vi "Write DateTime to Client.vi"(0 "OPC UA client refnum in":T1, 5 "Parent Node In":string, 7 "SubNode ID":string, 11 "error in (no error)":errorcluster, 12 "timestamp (current time)":timestamp) -> (4 "OPC UA client refnum out":T1, 6 "Parent Node Out":string, 15 "error out":errorcluster)   [LabVIEW 2024]
uses:
  <vilib>/OPCUA/controls/OPC UA Client Refnum.ctl
  <vilib>/OPCUA/controls/Write Status.ctl
  <vilib>/OPCUA/controls/NodeId.ctl
  <vilib>/OPCUA/client/Multiple Write DateTime.vi
  <vilib>/OPCUA/NI OPC UA Client.lvlib
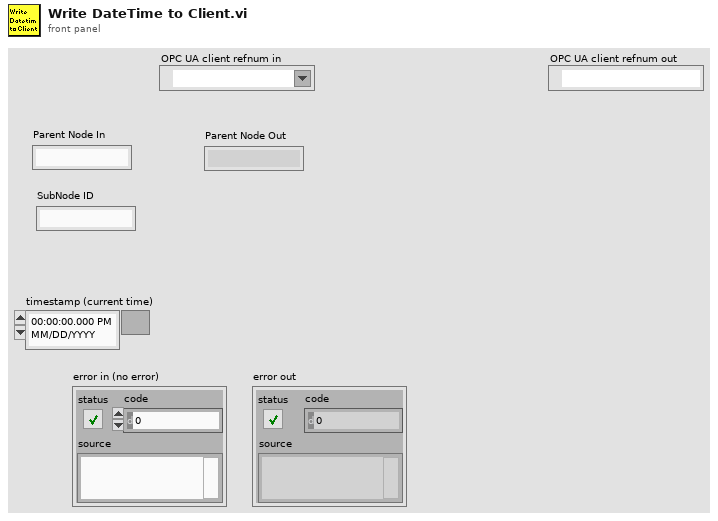
[diagram p1: front panel]
types:
  T1 = typedef "OPC UA Client Refnum.ctl" = refnum<k21>
  T2 = typedef "NodeId.ctl" = string
  T3 = typedef "Write Status.ctl" = u32
  T4 = cluster{"node ID":T2, "value":timestamp, "timestamp (current time)":timestamp, "node status":T3}
  T5 = cluster{"node ID":T2, "value":timestamp, "timestamp (current time)":timestamp, "node status":T3}[]
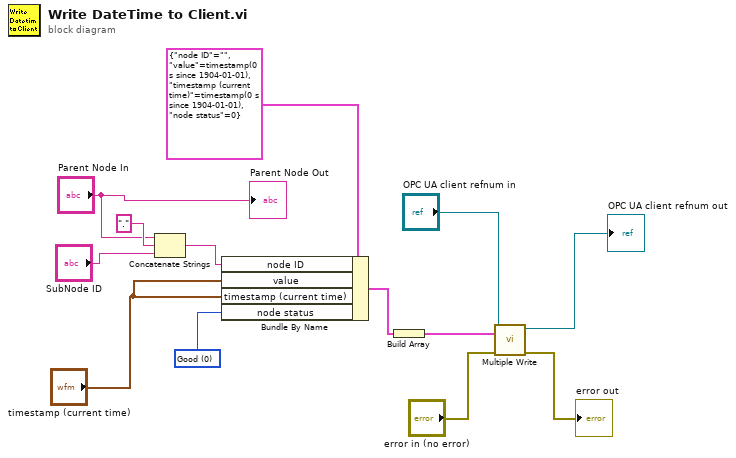
[diagram p0: block diagram]
diagram:
  w6 = T3 0 items=["Good"=0, "Uncertain"=1073741824, "Uncertain_InitialValue"=1083310080, "Uncertain_LastUsableValue"=1083179008, "Uncertain_SensorNotAccurate"=1083375616, "Uncertain_EngineeringUnitsExceeded"=1083441152, "Bad"=2147483648, "Bad_NoCommunication"=2150694912, "Bad_NotReadable"=2151284736, "Bad_NotWritable"=2151350272, "Bad_OutOfRange"=2151415808, "Bad_WaitingForInitialData"=2150760448] ("node status")
  n1 = Concatenate Strings("Parent Node In", ".", "SubNode ID") -> (w5:string)
  n2 = Bundle By Name(cluster=T4 {"node ID"="", "value"=timestamp(0 s since 1904-01-01), "timestamp (current time)"=timestamp(0 s since 1904-01-01), "node status"=0} ("request"), "node ID"=w5, "value"="timestamp (current time)", "timestamp (current time)"="timestamp (current time)", "node status"=w6) -> (w3:T4)
  n3 = Build Array(w3) -> (w2:T5)
  n4 = call-poly <vilib>:"Multiple Write.vi"("error in (no error)"="error in (no error)", "requests"=w2, "OPC UA client refnum in"="OPC UA client refnum in") -> ("error out"=→"error out":errorcluster, "OPC UA client refnum out"=→"OPC UA client refnum out":T1)  [unwired: 5 in, 2 out]
  "Parent Node Out" <- "Parent Node In"
